vi "WAPIAerClose.vi"(8 "error in (no error)":errorcluster, 11 "board":i16) -> (0 "error out":errorcluster)   [LabVIEW 2009]
uses:
  win50032.dll
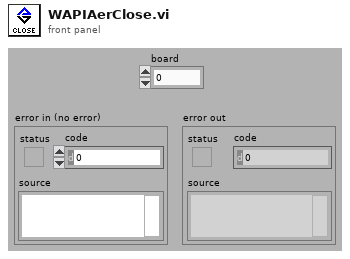
[diagram p1: front panel]
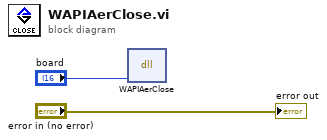
[diagram p0: block diagram]
diagram:
  n1 = dll-call lib="Win50032.dll" fn="WAPIAerClose"("board"="board") -> ()  [unwired: 5 in, 2 out]
  "error out" <- "error in (no error)"
